vi "Correct_Too_Long_Subtrack_with_Problems-1.vi"(4 "error IN":errorcluster, 5 "[IN] Minimal Subtrack Len\ngth for Making Desicion":i32, 6 "[IN] Status of problem point":i16, 7 "[IN] Subtracks":T1(array[cluster])) -> (0 "error OUT":errorcluster, 3 "[OUT] Subtracks":T1(array[cluster]))   [LabVIEW 2017]
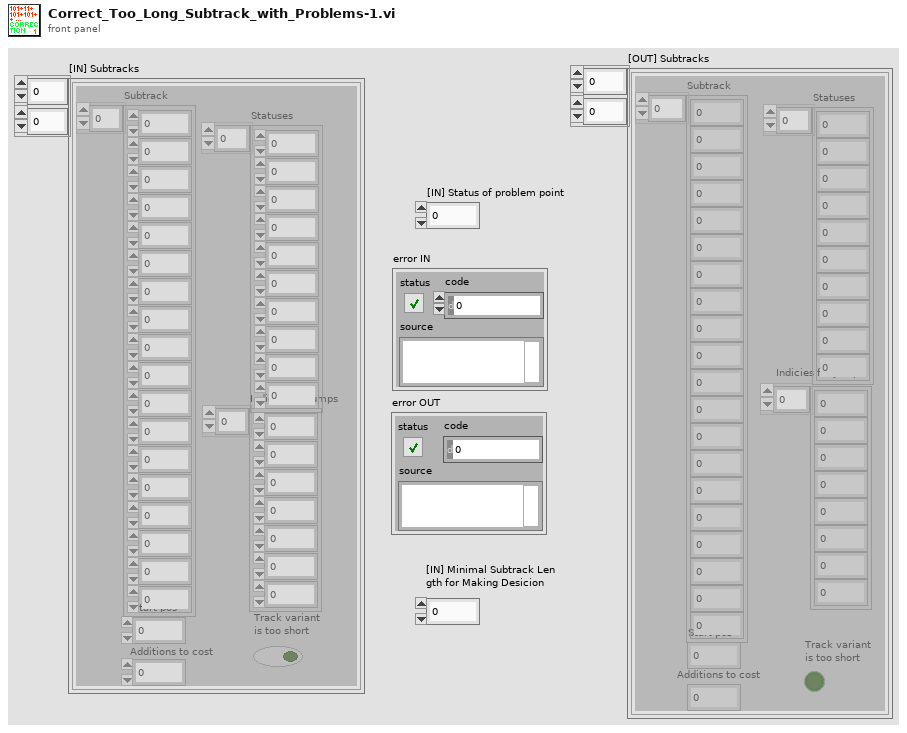
[diagram p1: front panel]
types:
  T1 = cluster{"Subtrack":dbl[], "Statuses":i16[], "Start pos":i32, "Additions to cost":i8, "Track variant \nis too short":bool, "Indicies for Jumps":i32[]}[][]
  T2 = cluster{"Subtrack":dbl[], "Statuses":i16[], "Start pos":i32, "Additions to cost":i8, "Track variant \nis too short":bool, "Indicies for Jumps":i32[]}[]
  T3 = cluster{"Subtrack":dbl[], "Statuses":i16[], "Start pos":i32, "Additions to cost":i8, "Track variant \nis too short":bool, "Indicies for Jumps":i32[]}
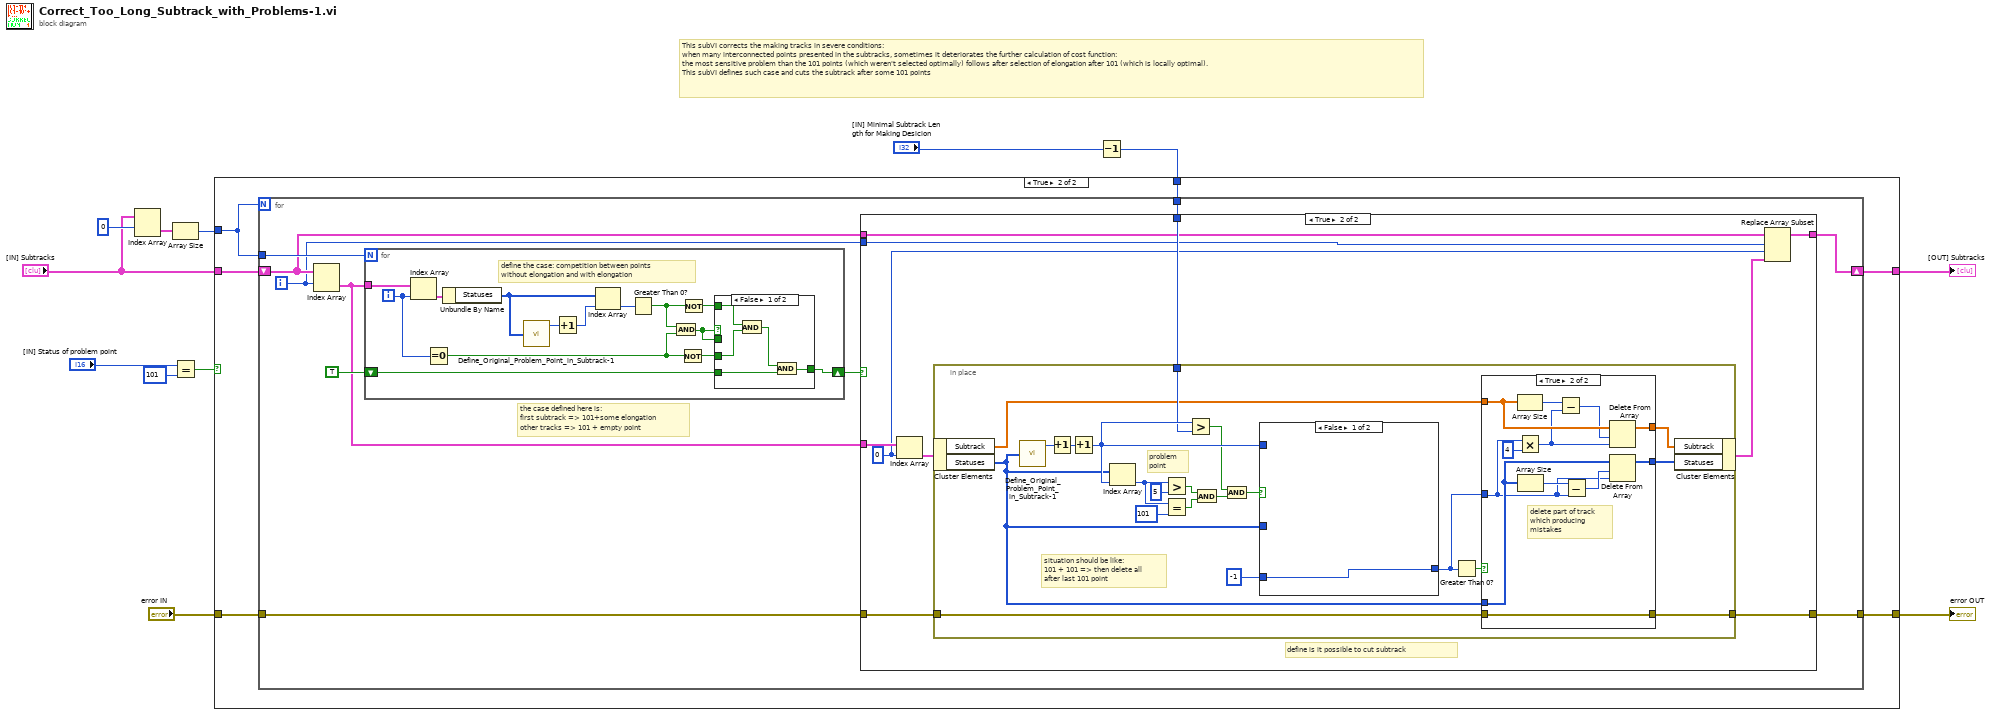
[diagram p0: block diagram]
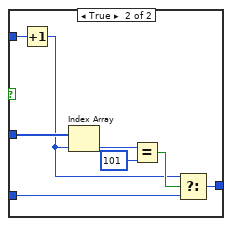
[diagram p5: hidden frame]
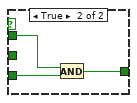
[diagram p6: hidden frame]
diagram:
  # "This subVI corrects the making tracks in severe conditions:\nwhen many interconnected points presented in the subtracks, sometimes it deteriorates the further calculation of cost function:\nthe most sensitive problem than the 101 points (which weren't selected optimally) follows after selection of elongation after 101 (which is locally optimal).\nThis subVI defines such case and cuts the subtrack after some 101 points"
  n1 = Index Array(array="[IN] Subtracks", index (row)=0) -> (element=w11:T2)  [unwired: 1 in]
  n2 = Array Size(array=w11) -> (size(s)=w10:i32)
  n3 = Equal?(x="[IN] Status of problem point", y=i16 101) -> (x = y?=w7:bool)
  n4 = Decrement(x="[IN] Minimal Subtrack Len\ngth for Making Desicion") -> (x-1=w4:i32)
  n5 = case shown="True" w7 {
    tunnel: w10 -> [_ w19]
    tunnel: "[IN] Subtracks" -> [w14 w20]
    tunnel: w4 -> [_ w18]
    tunnel: [w14 w17] -> w3
    tunnel: "error IN" -> [w13 w16]
    tunnel: [w13 w15] -> w1
    frame False {
    }
    frame True {
      n6 = for {
        N: w19 -> [_]
        tunnel: w19 -> [w30]
        shift-right: [w23] -> w17
        shift-left: w20 -> [w26]
        tunnel: w18 -> [w24]
        tunnel: w16 -> [w22]
        tunnel: [w21] -> w15
        i -> [w25]
        # "the case defined here is: \nfirst subtrack => 101+some elongation\nother tracks => 101 + empty point"
        n7 = Index Array(array=w26, index (row)=w25) -> (element=w27:T2)  [unwired: 1 in]
        n8 = for {
          N: w30 -> [_]
          tunnel: w27 -> [w101]
          shift-right: [w89] -> w28
          shift-left: TRUE -> [w94]
          i -> [w98]
          # "define the case: competition between points \nwithout elongation and with elongation"
          n9 = Index Array(array=w101, index=w98) -> (element=w99:T3)
          n10 = Equal To 0?(x=w98) -> (x = 0?=w93:bool)
          n11 = Unbundle By Name(w99) -> ("Statuses"=w97:i16[])
          n12 = call "Define_Original_Problem_Point_in_Subtrack-1.vi"("[IN] Statuses"=w97) -> ("[OUT] Index of Problem Point\nin Subtrack (Original)"=w100:i32)  [unwired: 3 in, 1 out]
          n13 = Increment(x=w100) -> (x+1=w96:i32)
          n14 = Index Array(array=w97, index=w96) -> (element=w95:i16)
          n15 = Greater Than 0?(x=w95) -> (x > 0?=w92:bool)
          n16 = And(x=w92, y=w93) -> (x .and. y?=w88:bool)
          n17 = Not(x=w93) -> (.not. x?=w90:bool)
          n18 = Not(x=w92) -> (.not. x?=w91:bool)
          n19 = case shown="False" w88 {
            tunnel: w94 -> [w104 w109]
            tunnel: [w102 w108] -> w89
            tunnel: w91 -> [w106 _]
            tunnel: w90 -> [w105 _]
            tunnel: w88 -> [_ w107]
            frame False {
              n20 = And(x=w106, y=w105) -> (x .and. y?=w103:bool)
              n21 = And(x=w103, y=w104) -> (x .and. y?=w102:bool)
            }
            frame True {
              n22 = And(x=w107, y=w109) -> (x .and. y?=w108:bool)
            }
          }
        }
        n23 = case shown="True" w28 {
          tunnel: w27 -> [_ w42]
          tunnel: w26 -> [w32 w39]
          tunnel: w25 -> [_ w38]
          tunnel: w24 -> [_ w40]
          tunnel: [w32 w35] -> w23
          tunnel: w22 -> [w31 w34]
          tunnel: [w31 w33] -> w21
          frame False {
          }
          frame True {
            w36 = 0
            # "define is it possible to cut subtrack"
            n24 = Index Array(array=w42, index=w36) -> (element=w41:T3)
            n25 = in-place {
              in-place-border: w40 -> [w60]
              in-place-border: w34 -> [w44]
              in-place-border: [w43] -> w33
              # "situation should be like: \n101 + 101 => then delete all\nafter last 101 point"
              # "problem \npoint"
              n26 = in-place-cluster #1(w41) -> ("Subtrack"=w46:dbl[], "Statuses"=w49:i16[])
              n27 = call "Define_Original_Problem_Point_in_Subtrack-1.vi"("[IN] Statuses"=w49) -> ("[OUT] Index of Problem Point\nin Subtrack (Original)"=w62:i32)  [unwired: 3 in, 1 out]
              n28 = Increment(x=w62) -> (x+1=w63:i32)
              n29 = Increment(x=w63) -> (x+1=w61:i32)
              n30 = Index Array(array=w49, index=w61) -> (element=w58:i16)
              n31 = Greater?(x=w58, y=i16 5) -> (0:w56:bool)
              n32 = Equal?(x=w58, y=i16 101) -> (x = y?=w55:bool)
              n33 = Greater?(x=w61, y=w60) -> (0:w53:bool)
              n34 = And(x=w56, y=w55) -> (x .and. y?=w54:bool)
              n35 = And(x=w53, y=w54) -> (x .and. y?=w52:bool)
              n36 = case shown="False" w52 {
                tunnel: w61 -> [_ w87]
                tunnel: w49 -> [_ w86]
                tunnel: -1 -> [w79 w80]
                tunnel: [w79 w82] -> w48
                frame False {
                }
                frame True {
                  n37 = Increment(x=w87) -> (x+1=w81:i32)
                  n38 = Index Array(array=w86, index=w81) -> (element=w84:i16)
                  n39 = Equal?(x=w84, y=i16 101) -> (x = y?=w83:bool)
                  n40 = Select(t=w81, s=w83, f=w80) -> (s? t:f=w82:i32)
                }
              }
              n41 = Greater Than 0?(x=w48) -> (x > 0?=w50:bool)
              n42 = case shown="True" w50 {
                tunnel: w49 -> [w65 w78]
                tunnel: w48 -> [_ w74]
                tunnel: [w65 w75] -> w47
                tunnel: w46 -> [w66 w72]
                tunnel: [w66 w68] -> w45
                tunnel: w44 -> [w64 w67]
                tunnel: [w64 w67] -> w43
                frame False {
                }
                frame True {
                  # "delete part of track\nwhich producing \nmistakes"
                  n43 = Array Size(array=w72) -> (size(s)=w71:i32)
                  n44 = Multiply(x=w74, y=4) -> (x*y=w70:i32)
                  n45 = Array Size(array=w78) -> (size(s)=w77:i32)
                  n46 = Subtract(x=w71, y=w70) -> (x-y=w69:i32)
                  n47 = Subtract(x=w77, y=w74) -> (x-y=w76:i32)
                  n48 = Delete From Array(array=w72, length=w69, index=w70) -> (array with subset deleted=w68:dbl[])  [unwired: 1 out]
                  n49 = Delete From Array(array=w78, length=w76, index=w74) -> (array with subset deleted=w75:i16[])  [unwired: 1 out]
                }
              }
              n50 = in-place-cluster #1("Subtrack"=w45, "Statuses"=w47) -> (w37:T3)
            }
            n51 = Replace Array Subset(array=w39, new element=w37, index (row)=w38, index (col)=w36) -> (w35:T1)
          }
        }
      }
    }
  }
  "error OUT" <- w1
  "[OUT] Subtracks" <- w3
